vi "Reshape volume imaging data.vi"(0 "tdms file ref":refnum<k34>, 1 "TDMS file path & name":path=path "C:/Users/Theo/Desktop/Datasets/140401_17_44_08-rig 3 debugging/Functional imaging TDMS data files/001.tdms", 5 "All header parameters":T1={"LOGIN"={"User"="Olympus  20X", "Profile"="", "Software Version"="", "Experiment Date Time"=timestamp(0 s since 1904-01-01)}, "GLOBAL PARAMETERS"={"MicroscopeID"="", "Microscope Type"="", "Objective"="", "Field of View (um)"=0.0, "Fill time (us)"=0.0, "Experiment Type"=enum."In vivo", "Stimuli Trigger"=FALSE, "Speed Logging"=FALSE}, "IMAGING MODES"={"Time Series"=FALSE, "Motor Zstack"=FALSE, "AOL Zstack"=FALSE, "Functional Imaging"=FALSE, "Volume Imaging"=FALSE}, "TIME SERIES"={"Basic Image meta data"={"Wavelength (nm)"=0.0, "# averaged frames"=0.0, "laser power (%)"=0.0, "Pockels"=0.0, "pixel dwell time (us)"=0.0, "pmt 1"=0.0, "pmt 2"=0.0, "back apperture"=0.0, "zoom"=0.0, "field of view"=0.0, "Frame Size"=0, "AOL x centre"=200.0, "AOL y centre"=0.0, "Stage x position"=0.0, "Stage y position"=0.0, "Stage z position"=0.0}, "AOL z"=0.0}, "MOTOR Z-STACK "={"Hdr Basic Image meta data"={"Wavelength (nm)"=0.0, "# averaged frames"=0.0, "laser power (%)"=0.0, "Pockels"=0.0, "pixel dwell time (us)"=0.0, "pmt 1"=0.0, "pmt 2"=0.0, "back apperture"=0.0, "zoom"=0.0, "field of view"=0.0, "Frame Size"=0, "AOL x centre"=0.0, "AOL y centre"=0.0, "Stage x position"=0.0, "Stage y position"=0.0, "Stage z position"=0.0}, "Z Start"=0.0, "Z Stop"=0.0, "No of Planes"=0, "Laser Power (%) at Z Start"=0.0, "Laser Power (%) at Z Stop"=0.0}, "AOL Z-STACK"={"Hdr Basic Image meta data"={"Wavelength (nm)"=0.0, "# averaged frames"=0.0, "laser power (%)"=0.0, "Pockels"=0.0, "pixel dwell time (us)"=0.0, "pmt 1"=0.0, "pmt 2"=0.0, "back apperture"=0.0, "zoom"=0.0, "field of view"=0.0, "Frame Size"=0, "AOL x centre"=0.0, "AOL y centre"=0.0, "Stage x position"=0.0, "Stage y position"=0.0, "Stage z position"=0.0}, "Z Start"=0.0, "Z Stop"=0.0, "No of Planes"=0, "Laser Power (%) at Z Start"=0.0, "Laser Power (%) at Z Stop"=0.0}, "FUNCTIONAL IMAGING"={"Functional Mode"=enum."Point", "Variable Length"=FALSE, "Variable Resolution"=FALSE, "Pockels Modulation"=FALSE, "Stimuli Trigger"=FALSE, "Cool down enabled"=FALSE, "AOL Mode"=enum."Raster", "Plane Mode"=0, "Miniscan Dwell time per pixel (us)"=0.0, "poi dwell time"=0.0, "Number of trials"=0.0, "Number of cycles"=0.0, "Number of pois"=0.0, "Number of miniscans"=0.0, "Number of pixels in miniscan"=0.0, "Rectangle ROI length"=0.0, "Rectangle ROI height"=0.0, "Frame rate (fps)"=0.0, "Acquisition Length"=0.0, "video length (sec)"=0.0, "Stimuli delay (sec)"=0.0, "Cool down time (sec)"=0.0, "Basic Image meta data"={"Wavelength (nm)"=0.0, "# averaged frames"=0.0, "laser power (%)"=0.0, "Pockels"=0.0, "pixel dwell time (us)"=0.0, "pmt 1"=0.0, "pmt 2"=0.0, "back apperture"=0.0, "zoom"=0.0, "field of view"=0.0, "Frame Size"=0, "AOL x centre"=0.0, "AOL y centre"=0.0, "Stage x position"=0.0, "Stage y position"=0.0, "Stage z position"=0.0}, "Z Start (um)"=0.0, "Z Stop (um)"=0.0}, "VOLUME IMAGING"={"Functional Mode"=enum."Point", "Variable Length"=FALSE, "Variable Resolution"=FALSE, "Pockels Modulation"=FALSE, "Stimuli Trigger"=FALSE, "Cool down enabled"=FALSE, "AOL Mode"=enum."Raster", "Plane Mode"=0, "Miniscan Dwell time per pixel (us)"=0.0, "poi dwell time"=0.0, "Number of trials"=0.0, "Number of cycles"=0.0, "Number of pois"=0.0, "Number of miniscans"=0.0, "Number of pixels in miniscan"=0.0, "Rectangle ROI length"=0.0, "Rectangle ROI height"=0.0, "Frame rate (fps)"=0.0, "Acquisition Length"=0.0, "video length (sec)"=0.0, "Stimuli delay (sec)"=0.0, "Cool down time (sec)"=0.0, "Basic Image meta data"={"Wavelength (nm)"=0.0, "# averaged frames"=0.0, "laser power (%)"=0.0, "Pockels"=0.0, "pixel dwell time (us)"=0.0, "pmt 1"=0.0, "pmt 2"=0.0, "back apperture"=0.0, "zoom"=0.0, "field of view"=0.0, "Frame Size"=0, "AOL x centre"=0.0, "AOL y centre"=0.0, "Stage x position"=0.0, "Stage y position"=0.0, "Stage z position"=0.0}, "Z Start (um)"=0.0, "Z Stop (um)"=0.0}, "MOVEMENT CORRECTION"={"Movement Correction"=FALSE, "Axial Reference"=FALSE, "Reference Source"=enum."Green channel", "Full Frame Size"=0.0, "Reference Field of View"=0.0, "Reference Zoom"=0.0, "Reference dwell time (us)"=0.0, "Reference X Pixels"=0.0, "Reference Y Pixels"=0.0, "Number of Z lines"=0.0, "Size of Z pixels"=0.0, "Axial Pixels"=0.0, "Ignore Z lines"=0.0, "Reference Scan Cycles"=0.0, "Reference Threshold XY"=0.0, "Reference Threshold Z"=0.0, "Reference Average XY"=0.0, "Reference Average Z"=0.0, "Proportional Scale"=0.0, "Integral Scale"=0.0, "Proportional Scale Z"=0.0, "Integral Scale Z"=0.0, "Diff Threshold"=0.0, "Diff Threshold Z"=0.0, "Sliding Average"=FALSE, "Reference count reset enabled"=FALSE, "Scan Interval (ms)"=0.0, "Ref Plot Refresh Rate (ms)"=0.0}, "CALIBRATION"={"Pockels Calibration File"=path "", "Calibration_ini file"=path "", "Setup_ini file"=path ""}, "STATISTICS"={"Z-stack duration (sec)"=0.0, "Number of acquired data-points"=0.0, "Acquisition time (ms)"=0.0, "Number of acquired frames"=0.0, "Intertrial times"=[]}, "BIOLOGY INFORMATION"={"Animal Code or Name"="", "Animal DoB"="", "Animal Age"="", "Animal Sex"="", "Animal Weight"="", "Date of Injection"="", "Date of Implant"="", "Site of Injection"="", "Animal Ear Notch"="", "AAV constructs"="", "Genetic background"="", "Optical reporter"="", "Region of brain imaged"="", "Other \ncomments"=""}, "Calibration Data"={"Objective Name"="", "Calibration Wavelength"=0.0, "Sum X"=0.0, "Sum Y"=0.0, "Diff X"=0.0, "Diff Y"=0.0, "Distortion Correction"=0.0, " Z norm to um Scaling"=0.0, " X norm to um Scaling"=0.0}} {"VOLUME IMAGING"."Plane Mode" items=["XY Plane", "XZ Plane", "YZ Plane", "arbitraryplane"]; "VOLUME IMAGING"."Basic Image meta data"."Frame Size" items=["100X100"=100, "128X128"=128, "200X200"=200, "256X256"=256, "512X512"=512, "1024x1024"=1024, "2048x2048"=2048]; "AOL Z-STACK"."Hdr Basic Image meta data"."Frame Size" items=["100X100"=100, "128X128"=128, "200X200"=200, "256X256"=256, "512X512"=512, "1024x1024"=1024, "2048x2048"=2048]; "MOTOR Z-STACK"."Hdr Basic Image meta data"."Frame Size" items=["100X100"=100, "128X128"=128, "200X200"=200, "256X256"=256, "512X512"=512, "1024x1024"=1024, "2048x2048"=2048]; "FUNCTIONAL IMAGING"."Plane Mode" items=["XY Plane", "XZ Plane", "YZ Plane", "arbitraryplane"]; "FUNCTIONAL IMAGING"."Basic Image meta data"."Frame Size" items=["100X100"=100, "128X128"=128, "200X200"=200, "256X256"=256, "512X512"=512, "1024x1024"=1024, "2048x2048"=2048]; "TIME SERIES"."Basic Image meta data"."Frame Size" items=["100X100"=100, "128X128"=128, "200X200"=200, "256X256"=256, "512X512"=512, "1024x1024"=1024, "2048x2048"=2048]}, 11 "error in (no error)":errorcluster, 12 "Channel to process":enum16{"Red", "Green", "Both"}(ring)) -> (4 "tdms file out":refnum<k34>, 6 "Single channel data":u16[](array[numeric]), 8 "Channel 4D data":u16[][][][](array[numeric]), 10 "Volumetric parameters":T21, 14 "Angles (deg)":dbl[](array[numeric]), 15 "error out":errorcluster)   [LabVIEW 2020]
uses:
  User Interface/Visualisation/Functional Imaging Viewer/SubVIs/Experiment header interface/Typedefs/Header parameters cluster-ALL.ctl
  User Interface/Visualisation/Functional Imaging Viewer/SubVIs/Experiment header interface/Typedefs/Header subclusters/Header params -Login.ctl
  User Interface/Visualisation/Functional Imaging Viewer/SubVIs/Experiment header interface/Typedefs/Header subclusters/Header params-Global Parameters.ctl
  User Interface/Misc/Experiment Type.ctl
  User Interface/Visualisation/Functional Imaging Viewer/SubVIs/Experiment header interface/Typedefs/Header subclusters/Header params-Imaging Modes.ctl
  User Interface/Visualisation/Functional Imaging Viewer/SubVIs/Experiment header interface/Typedefs/Header subclusters/Header params-Time Series.ctl
  User Interface/Visualisation/Functional Imaging Viewer/SubVIs/Experiment header interface/Typedefs/Header subclusters/Header params-Basic image meta data.ctl
  Typedefs/Frame Size.ctl
  User Interface/Visualisation/Functional Imaging Viewer/SubVIs/Experiment header interface/Typedefs/Header subclusters/Header params-Motor Z-stack.ctl
  User Interface/Visualisation/Functional Imaging Viewer/SubVIs/Experiment header interface/Typedefs/Header subclusters/Header params-AOL Z-stack.ctl
  User Interface/Visualisation/Functional Imaging Viewer/SubVIs/Experiment header interface/Typedefs/Header subclusters/Header params-Functional Imaging.ctl
  Typedefs/Functional Mode.ctl
  Typedefs/AOL modes.ctl
  Typedefs/Plane Mode.ctl
  User Interface/Visualisation/Functional Imaging Viewer/SubVIs/Experiment header interface/Typedefs/Header subclusters/Header params-Movement correction.ctl
  Typedefs/Reference source.ctl
  User Interface/Visualisation/Functional Imaging Viewer/SubVIs/Experiment header interface/Typedefs/Header subclusters/Header params-Calibration Setup.ctl
  User Interface/Visualisation/Functional Imaging Viewer/SubVIs/Experiment header interface/Typedefs/Header subclusters/Header params-statistics.ctl
  User Interface/Misc/Biology Information.ctl
  User Interface/Visualisation/Functional Imaging Viewer/SubVIs/Experiment header interface/Typedefs/Header subclusters/Header params-calibration data.ctl
panel:
  in  "Channel to process":enum16{"Red", "Green"}(ring)
  out "Points in each volume or trial (fractional)":dbl
  out "Points Mismatch":bool
  out "Resulting number of points":i32
  out "Points in each volume or trial":i32
  out "Points in all volumes":i32
  out "Channel size(s)":i32[](array[numeric])
  # "<---This should be an integer. If it is not review the logic inside this VI is suitable"
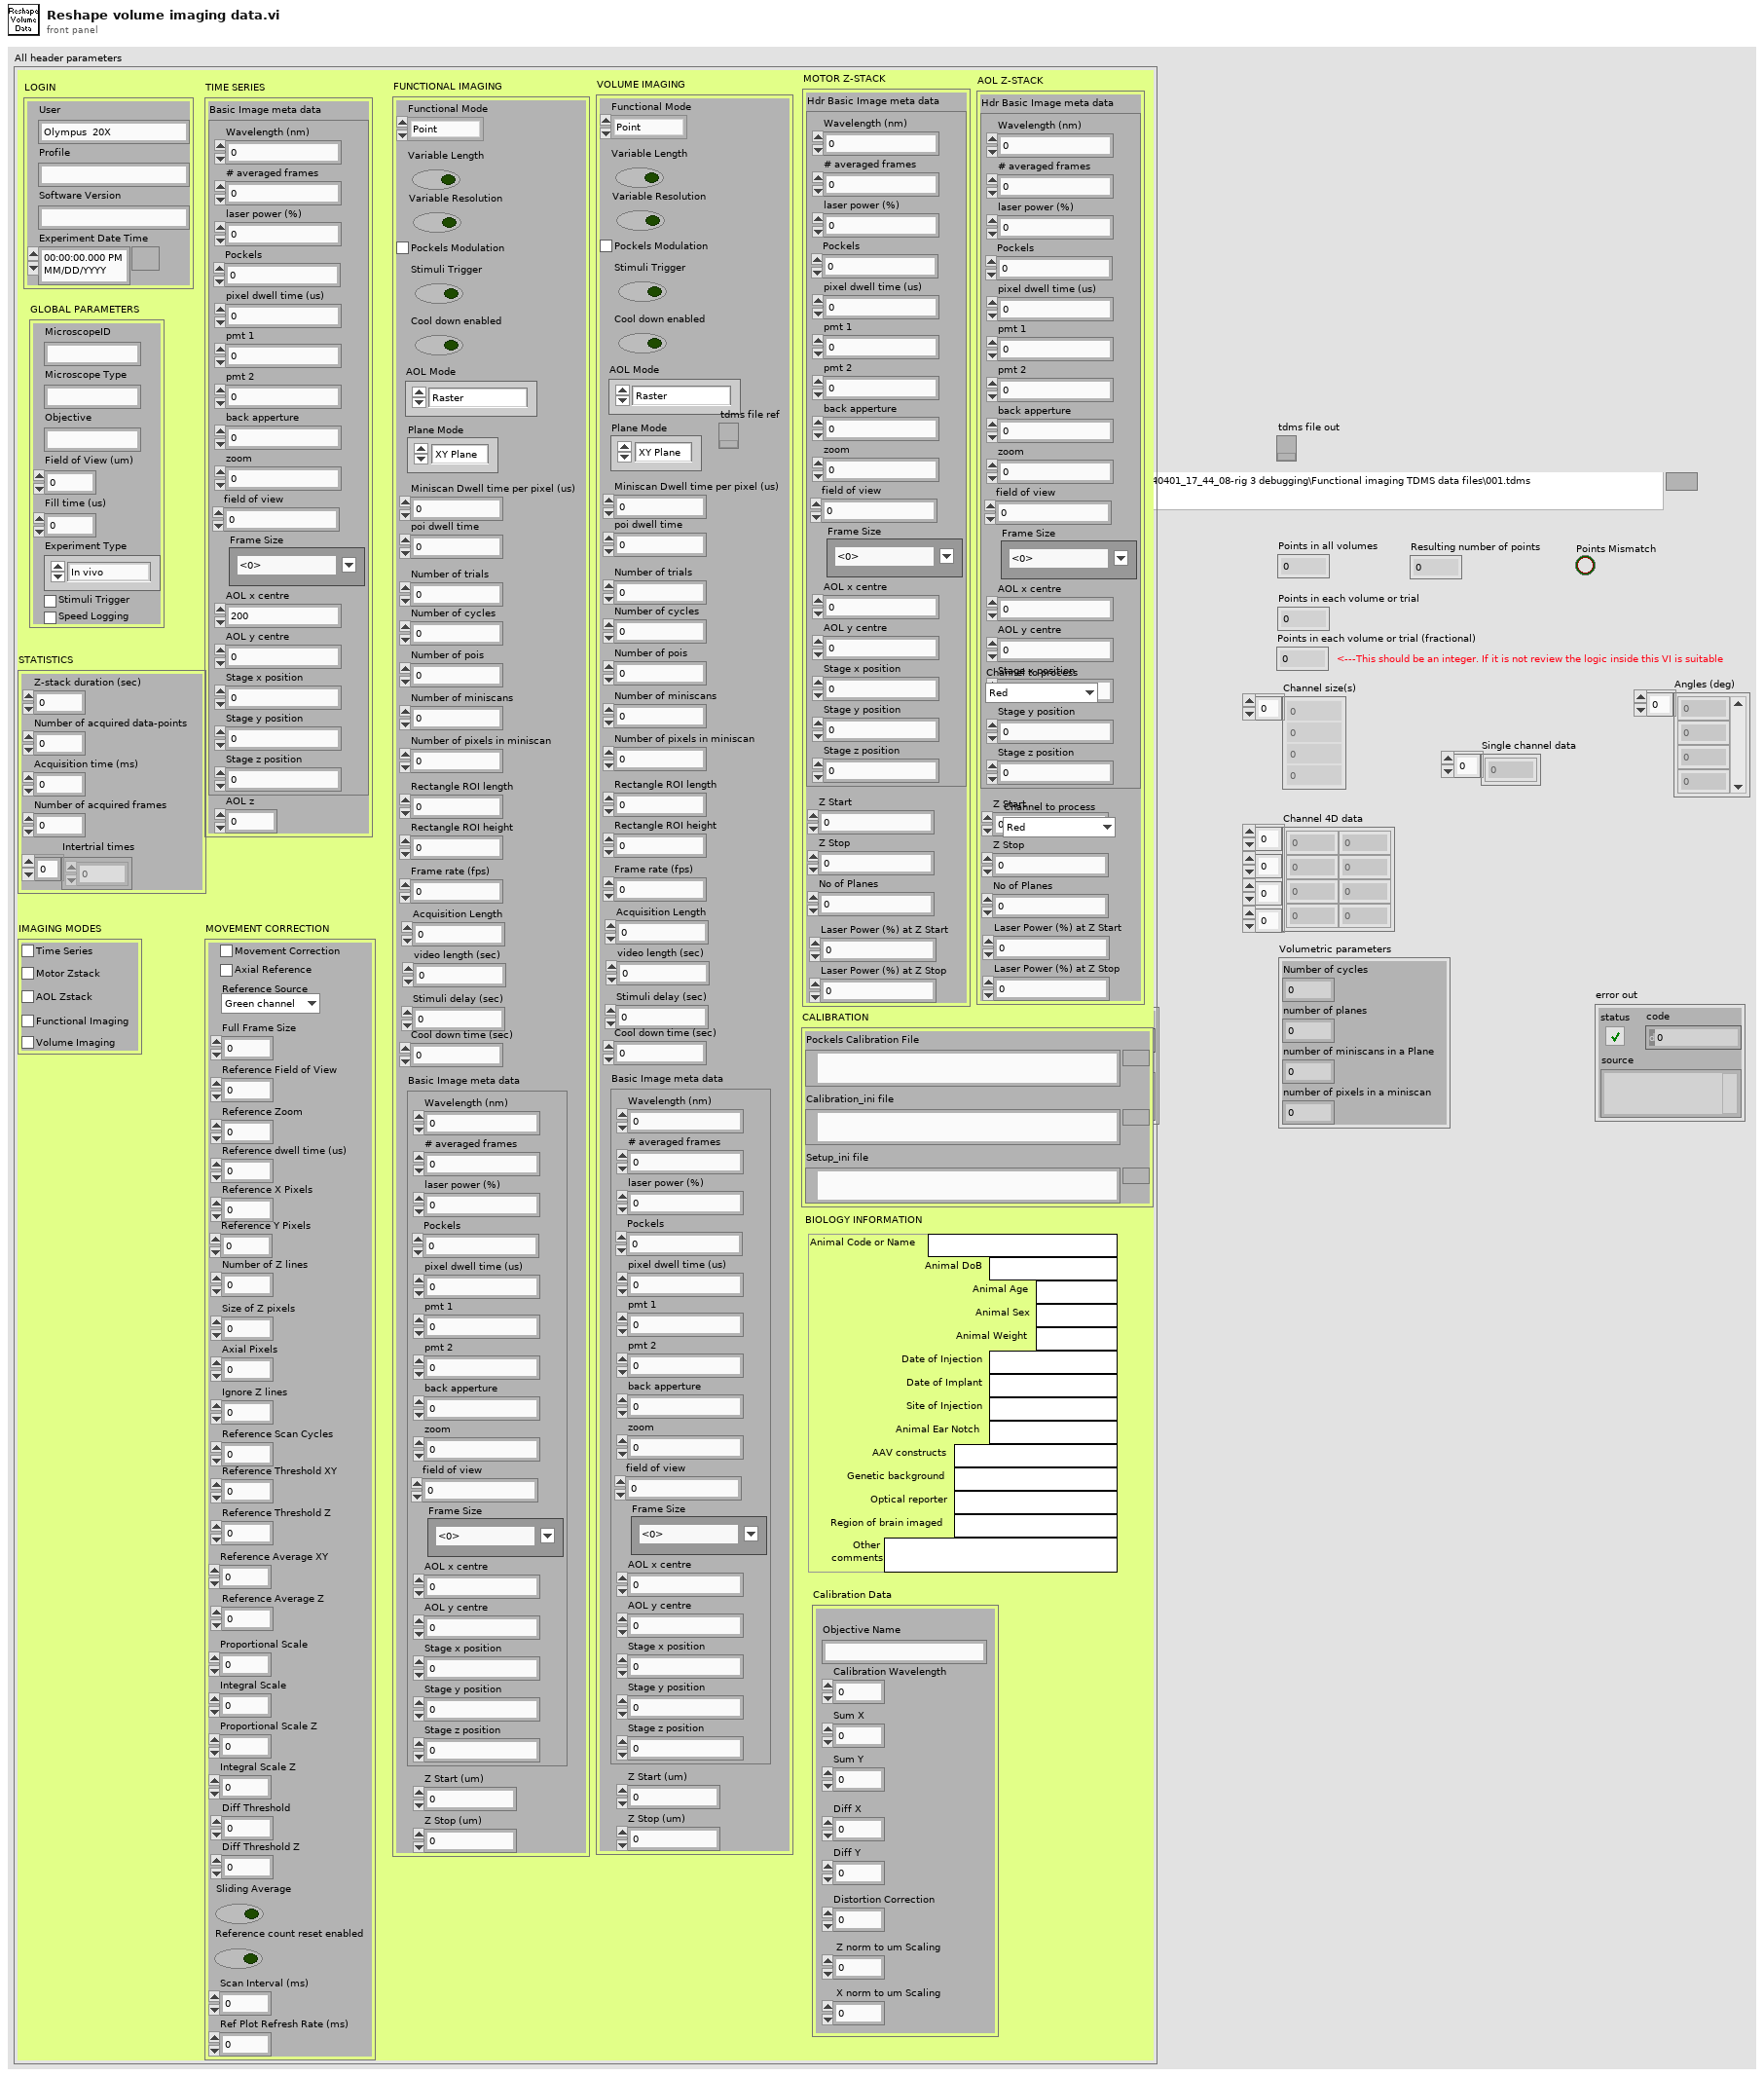
[diagram p1: front panel]
types:
  T1 = typedef "Header parameters cluster-ALL.ctl" = cluster{"LOGIN":T2, "GLOBAL PARAMETERS":T3, "IMAGING MODES":T5, "TIME SERIES":T6, "MOTOR Z-STACK ":T9, "AOL Z-STACK":T10, "FUNCTIONAL IMAGING":T11, "VOLUME IMAGING":T11, "MOVEMENT CORRECTION":T15, "CALIBRATION":T17, "STATISTICS":T18, "BIOLOGY INFORMATION":T19, "Calibration Data":T20}
  T2 = typedef "Header params -Login.ctl" = cluster{"User":string, "Profile":string, "Software Version":string, "Experiment Date Time":timestamp}
  T3 = typedef "Header params-Global Parameters.ctl" = cluster{"MicroscopeID":string, "Microscope Type":string, "Objective":string, "Field of View (um)":dbl, "Fill time (us)":dbl, "Experiment Type":T4, "Stimuli Trigger":bool, "Speed Logging":bool}
  T4 = typedef "Experiment Type.ctl" = enum16{"In vivo", "In vitro", "Testing", "Calibration", "Other"}
  T5 = typedef "Header params-Imaging Modes.ctl" = cluster{"Time Series":bool, "Motor Zstack":bool, "AOL Zstack":bool, "Functional Imaging":bool, "Volume Imaging":bool}
  T6 = typedef "Header params-Time Series.ctl" = cluster{"Basic Image meta data":T7, "AOL z":dbl}
  T7 = typedef "Header params-Basic image meta data.ctl" = cluster{"Wavelength (nm)":dbl, "# averaged frames":dbl, "laser power (%)":dbl, "Pockels":dbl, "pixel dwell time (us)":dbl, "pmt 1":dbl, "pmt 2":dbl, "back apperture":dbl, "zoom":dbl, "field of view":dbl, "Frame Size":T8, "AOL x centre":dbl, "AOL y centre":dbl, "Stage x position":dbl, "Stage y position":dbl, "Stage z position":dbl}
  T8 = typedef "Frame Size.ctl" = u16
  T9 = typedef "Header params-Motor Z-stack.ctl" = cluster{"Hdr Basic Image meta data":T7, "Z Start":dbl, "Z Stop":dbl, "No of Planes":i32, "Laser Power (%) at Z Start":dbl, "Laser Power (%) at Z Stop":dbl}
  T10 = typedef "Header params-AOL Z-stack.ctl" = cluster{"Hdr Basic Image meta data":T7, "Z Start":dbl, "Z Stop":dbl, "No of Planes":i32, "Laser Power (%) at Z Start":dbl, "Laser Power (%) at Z Stop":dbl}
  T11 = typedef "Header params-Functional Imaging.ctl" = cluster{"Functional Mode":T12, "Variable Length":bool, "Variable Resolution":bool, "Pockels Modulation":bool, "Stimuli Trigger":bool, "Cool down enabled":bool, "AOL Mode":T13, "Plane Mode":T14, "Miniscan Dwell time per pixel (us)":dbl, "poi dwell time":dbl, "Number of trials":dbl, "Number of cycles":dbl, "Number of pois":dbl, "Number of miniscans":dbl, "Number of pixels in miniscan":dbl, "Rectangle ROI length":dbl, "Rectangle ROI height":dbl, "Frame rate (fps)":dbl, "Acquisition Length":dbl, "video length (sec)":dbl, "Stimuli delay (sec)":dbl, "Cool down time (sec)":dbl, "Basic Image meta data":T7, "Z Start (um)":dbl, "Z Stop (um)":dbl}
  T12 = typedef "Functional Mode.ctl" = enum16{"Point", "Line", "Patch", "Plane", "Volume"}
  T13 = typedef "AOL modes.ctl" = enum16{"Raster", "Structural", "Pointing", "Mini Scan", "Alignment"}
  T14 = typedef "Plane Mode.ctl" = u16
  T15 = typedef "Header params-Movement correction.ctl" = cluster{"Movement Correction":bool, "Axial Reference":bool, "Reference Source":T16, "Full Frame Size":dbl, "Reference Field of View":dbl, "Reference Zoom":dbl, "Reference dwell time (us)":dbl, "Reference X Pixels":dbl, "Reference Y Pixels":dbl, "Number of Z lines":dbl, "Size of Z pixels":dbl, "Axial Pixels":dbl, "Ignore Z lines":dbl, "Reference Scan Cycles":dbl, "Reference Threshold XY":dbl, "Reference Threshold Z":dbl, "Reference Average XY":dbl, "Reference Average Z":dbl, "Proportional Scale":dbl, "Integral Scale":dbl, "Proportional Scale Z":dbl, "Integral Scale Z":dbl, "Diff Threshold":dbl, "Diff Threshold Z":dbl, "Sliding Average":bool, "Reference count reset enabled":bool, "Scan Interval (ms)":dbl, "Ref Plot Refresh Rate (ms)":dbl}
  T16 = typedef "Reference source.ctl" = enum16{"Green channel", "Red channel"}
  T17 = typedef "Header params-Calibration Setup.ctl" = cluster{"Pockels Calibration File":path, "Calibration_ini file":path, "Setup_ini file":path}
  T18 = typedef "Header params-statistics.ctl" = cluster{"Z-stack duration (sec)":dbl, "Number of acquired data-points":dbl, "Acquisition time (ms)":dbl, "Number of acquired frames":dbl, "Intertrial times":dbl[]}
  T19 = typedef "Biology Information.ctl" = cluster{"Animal Code or Name":string, "Animal DoB":string, "Animal Age":string, "Animal Sex":string, "Animal Weight":string, "Date of Injection":string, "Date of Implant":string, "Site of Injection":string, "Animal Ear Notch":string, "AAV constructs":string, "Genetic background":string, "Optical reporter":string, "Region of brain imaged":string, "Other \ncomments":string}
  T20 = typedef "Header params-calibration data.ctl" = cluster{"Objective Name":string, "Calibration Wavelength":dbl, "Sum X":dbl, "Sum Y":dbl, "Diff X":dbl, "Diff Y":dbl, "Distortion Correction":dbl, " Z norm to um Scaling":dbl, " X norm to um Scaling":dbl}
  T21 = cluster{"Number of cycles":i32, "number of planes":i32, "number of miniscans in a Plane":i32, "number of pixels in a miniscan":i32}
  T22 = cluster{"Number of trials/volumes":i32, "number of planes":i32, "number of miniscans in a Plane":i32, "number of pixels in a miniscan":i32}
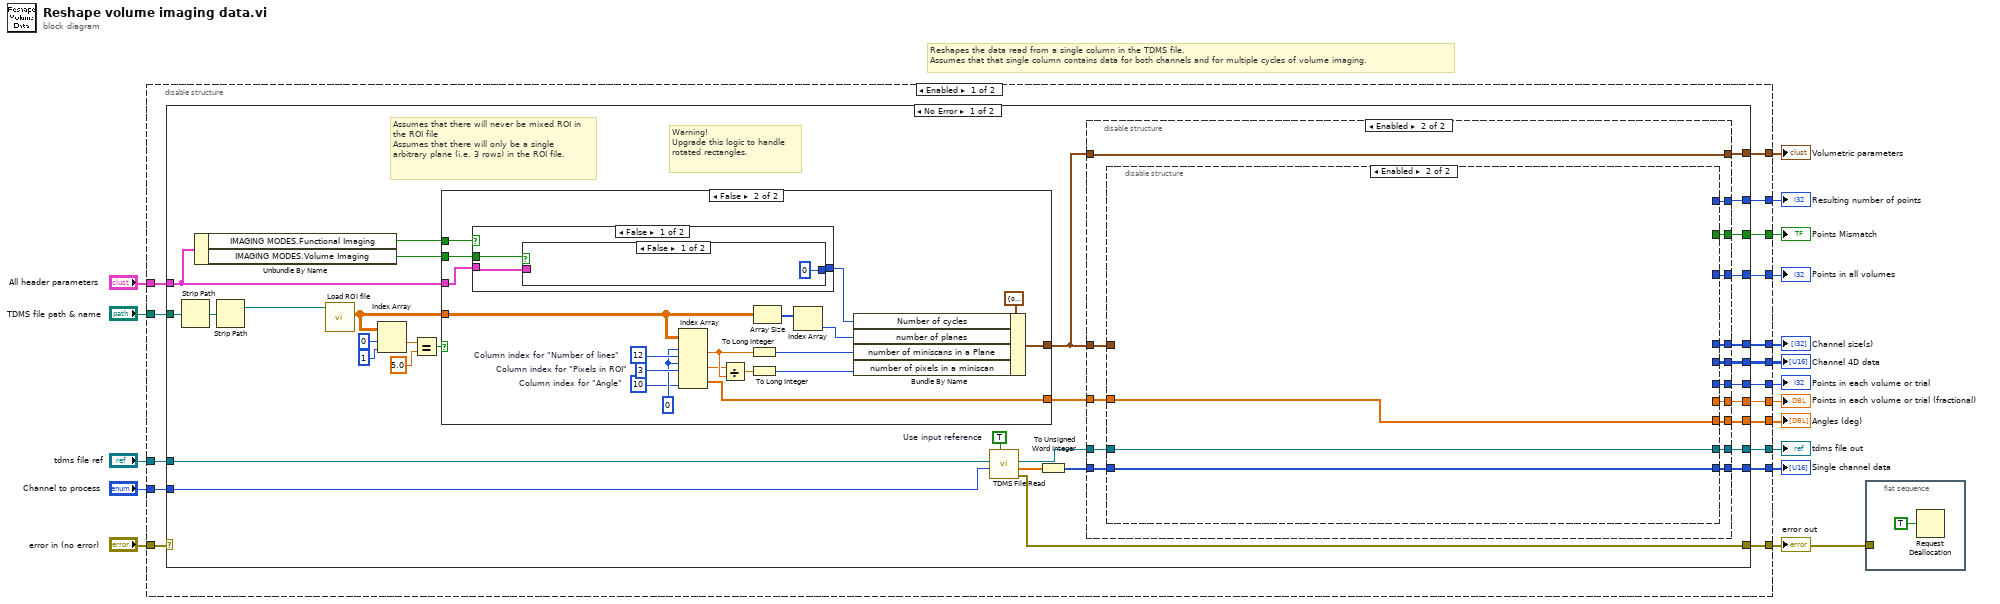
[diagram p0: block diagram]
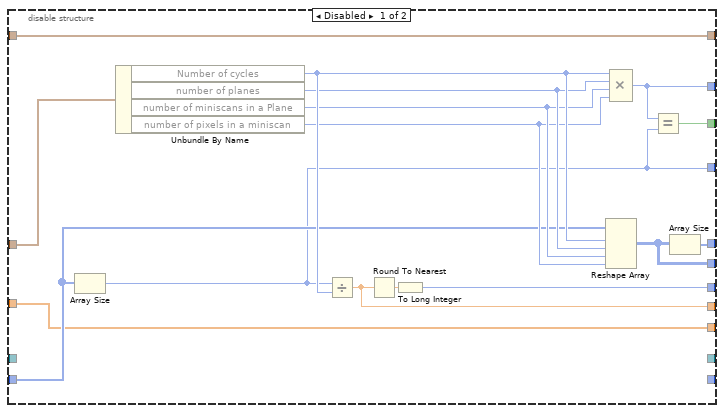
[diagram p2: hidden frame]
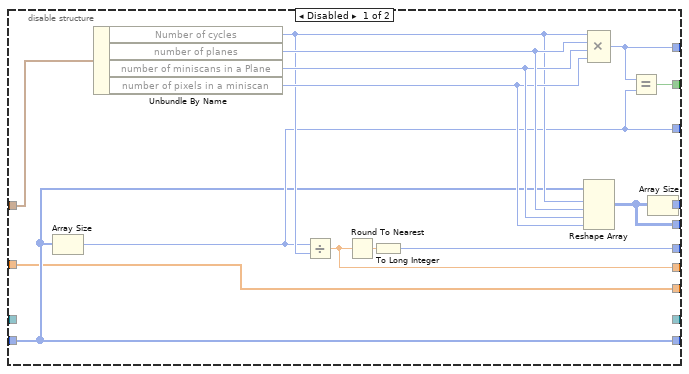
[diagram p3: hidden frame]
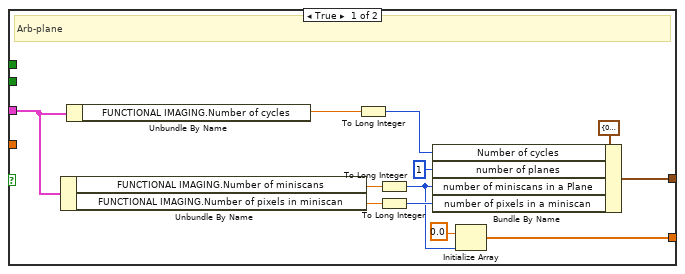
[diagram p4: hidden frame]
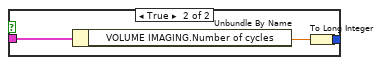
[diagram p5: hidden frame]
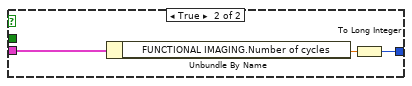
[diagram p6: hidden frame]
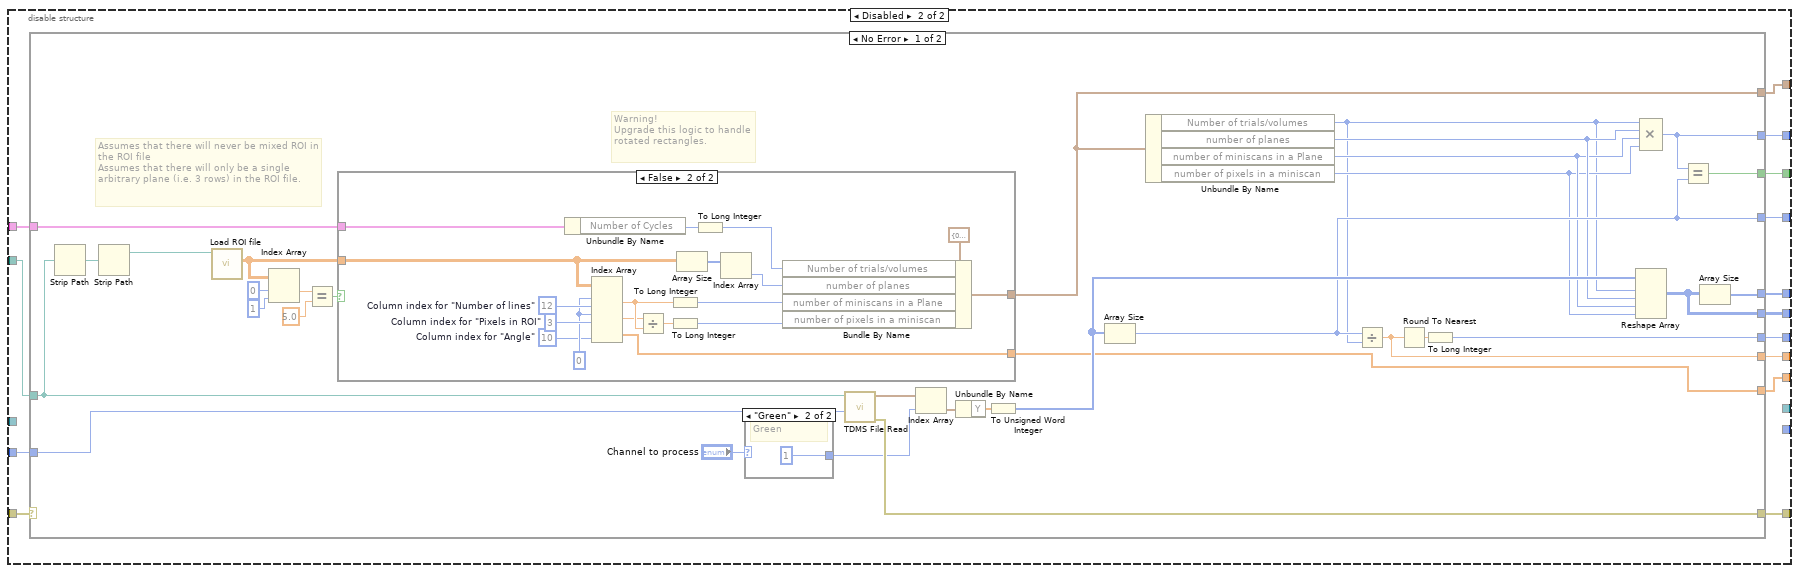
[diagram p8: hidden frame]
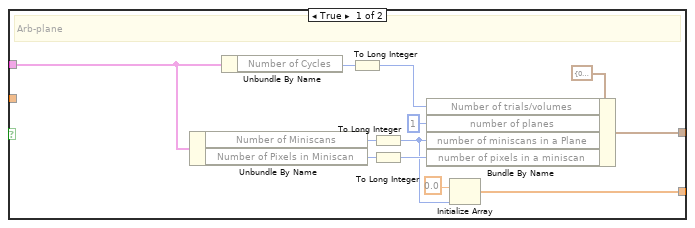
[diagram p9: hidden frame]
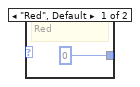
[diagram p10: hidden frame]
diagram:
  # "Reshapes the data read from a single column in the TDMS file.\nAssumes that that single column contains data for both channels and for multiple cycles of volume imaging."
  n1 = disable-structure shown="Enabled" {
    disable-tunnel: [w34 w171] -> w17
    disable-tunnel: "TDMS file path & name" -> [w33 w170]
    disable-tunnel: [w32 w169] -> w15
    disable-tunnel: [w31 w168] -> w14
    disable-tunnel: [w30 w167] -> w13
    disable-tunnel: "error in (no error)" -> [w29 w166]
    disable-tunnel: [w28 w165] -> w11
    disable-tunnel: [w27 w164] -> w10
    disable-tunnel: [w26 w163] -> w9
    disable-tunnel: "All header parameters" -> [w25 w162]
    disable-tunnel: [w24 w161] -> w7
    disable-tunnel: [w23 w160] -> w6
    disable-tunnel: [w22 w159] -> w5
    disable-tunnel: "Channel to process" -> [w21 w158]
    disable-tunnel: [w20 _] -> w3
    disable-tunnel: "tdms file ref" -> [w19 _]
    disable-tunnel: [w18 _] -> w1
    frame Enabled {
      n2 = case shown="No Error" w29 {
        selector: w29 -> [_ w157]
        tunnel: [w66 _] -> w34
        tunnel: w33 -> [w60 _]
        tunnel: [w65 _] -> w32
        tunnel: [w64 _] -> w31
        tunnel: [w63 _] -> w30
        tunnel: [w59 w157] -> w28
        tunnel: w25 -> [w37 _]
        tunnel: [w43 _] -> w26
        tunnel: [w47 _] -> w27
        tunnel: [w51 _] -> w24
        tunnel: [w50 _] -> w23
        tunnel: [w49 _] -> w22
        tunnel: w21 -> [w46 _]
        tunnel: [w45 _] -> w20
        tunnel: w19 -> [w41 _]
        tunnel: [w38 _] -> w18
        frame No Error {
          w42 = TRUE  # Use input reference
          # "Assumes that there will never be mixed ROI in the ROI file\nAssumes that there will only be a single arbitrary plane (i.e. 3 rows) in the ROI file."
          # "Warning!\nUpgrade this logic to handle rotated rectangles."
          n3 = Strip Path(path=w60) -> (stripped path=w61:path)  [unwired: 1 out]
          n4 = Unbundle By Name(w37) -> ("IMAGING MODES.Functional Imaging"=w36:bool, "IMAGING MODES.Volume Imaging"=w35:bool)
          n5 = Strip Path(path=w61) -> (stripped path=w62:path)  [unwired: 1 out]
          n6 = call "Load ROI file.vi"("Experiment data folder path"=w62) -> ("ROI Data (header removed)"=w58:dbl[][])  [unwired: 7 in, 3 out]
          n7 = Index Array(array=w58, index (row)=0, index (col)=1 ("disabled index (col)")) -> (element=w55:dbl)
          n8 = Equal?(x=w55, y=5.0) -> (x = y?=w53:bool)
          n9 = case shown="False" w53 {
            tunnel: [w127 w142] -> w44
            tunnel: [w123 w133] -> w48
            tunnel: w58 -> [_ w134]
            tunnel: w37 -> [w119 w131]
            tunnel: w36 -> [_ w129]
            tunnel: w35 -> [_ w128]
            frame True {
              # "Arb-plane"
              n10 = Unbundle By Name(w119) -> ("FUNCTIONAL IMAGING.Number of miniscans"=w118:dbl, "FUNCTIONAL IMAGING.Number of pixels in miniscan"=w117:dbl)
              n11 = Unbundle By Name(w119) -> ("FUNCTIONAL IMAGING.Number of cycles"=w121:dbl)
              n12 = To Long Integer(number=w121) -> (32bit integer=w120:i32)
              n13 = To Long Integer(number=w118) -> (32bit integer=w122:i32)
              n14 = To Long Integer(number=w117) -> (32bit integer=w125:i32)
              n15 = Bundle By Name(cluster=T21 {"Number of cycles"=0, "number of planes"=0, "number of miniscans in a Plane"=0, "number of pixels in a miniscan"=0} ("Parameters Cluster"), "Number of cycles"=w120, "number of planes"=1, "number of miniscans in a Plane"=w122, "number of pixels in a miniscan"=w125) -> (w127:T21)
              n16 = Initialize Array(0.0 ("element"), w122) -> (w123:dbl[])
            }
            frame False {
              w139 = 10  # Column index for "Angle"
              w140 = 0 ("disabled index (row)")
              w145 = 3  # Column index for "Pixels in ROI"
              w146 = 12  # Column index for "Number of lines"
              n17 = case shown="False" w129 {
                tunnel: [w148 w155] -> w132
                tunnel: w131 -> [w149 w154]
                tunnel: w128 -> [w147 _]
                frame False {
                  n18 = case shown="False" w147 {
                    tunnel: w149 -> [_ w152]
                    tunnel: [0 w151] -> w148
                    frame False {
                    }
                    frame True {
                      n19 = Unbundle By Name(w152) -> ("VOLUME IMAGING.Number of cycles"=w153:dbl)
                      n20 = To Long Integer(number=w153) -> (32bit integer=w151:i32)
                    }
                  }
                }
                frame True {
                  n21 = Unbundle By Name(w154) -> ("FUNCTIONAL IMAGING.Number of cycles"=w156:dbl)
                  n22 = To Long Integer(number=w156) -> (32bit integer=w155:i32)
                }
              }
              n23 = Index Array(array=w134, index (row) #1=w140, index (col) #1=w146, index (row) #2=w140, index (col) #2=w145, index (col) #3=w139) -> (element #1=w138:dbl, element #2=w137:dbl, element #3=w133:dbl[])  [unwired: 1 in]
              n24 = Divide(x=w137, y=w138) -> (x/y=w141:dbl)
              n25 = To Long Integer(number=w138) -> (32bit integer=w136:i32)
              n26 = To Long Integer(number=w141) -> (32bit integer=w135:i32)
              n27 = Array Size(array=w134) -> (size(s)=w144:i32[])
              n28 = Index Array(array=w144) -> (element=w143:i32)  [unwired: 1 in]
              n29 = Bundle By Name(cluster=T21 {"Number of cycles"=0, "number of planes"=0, "number of miniscans in a Plane"=0, "number of pixels in a miniscan"=0} ("Parameters Cluster"), "Number of cycles"=w132, "number of planes"=w143, "number of miniscans in a Plane"=w136, "number of pixels in a miniscan"=w135) -> (w142:T21)
            }
          }
          n30 = call "TDMS File Read.vi"("Use input reference (F)"=w42, "Channel to load"=w46, "tdms file ref"=w41) -> ("Error Out"=w59:errorcluster, "Single channel data"=w40:dbl[], "tdms file out"=w39:refnum<k34>)  [unwired: 4 in, 2 out]
          n31 = To Unsigned Word Integer(number=w40) -> (unsigned 16bit integer=w52:u16[])
          n32 = disable-structure shown="Enabled" {
            disable-tunnel: [w82 w97] -> w66
            disable-tunnel: [w80 w96] -> w65
            disable-tunnel: [w79 w95] -> w64
            disable-tunnel: [w78 w94] -> w63
            disable-tunnel: w44 -> [w67 w90]
            disable-tunnel: w52 -> [w73 w89]
            disable-tunnel: [w72 w93] -> w51
            disable-tunnel: [w71 w92] -> w50
            disable-tunnel: [w70 w91] -> w49
            disable-tunnel: w48 -> [w69 w87]
            disable-tunnel: [w69 w86] -> w47
            disable-tunnel: [_ w88] -> w45
            disable-tunnel: w44 -> [w68 w85]
            disable-tunnel: [w68 w85] -> w43
            disable-tunnel: w39 -> [_ w84]
            disable-tunnel: [_ w83] -> w38
            frame Disabled {
              n33 = Array Size(array=w73) -> (size(s)=w70:i32)
              n34 = Unbundle By Name(w67) -> ("Number of cycles"=w77:i32, "number of planes"=w76:i32, "number of miniscans in a Plane"=w75:i32, "number of pixels in a miniscan"=w74:i32)
              n35 = Divide(x=w70, y=w77) -> (x/y=w71:dbl)
              n36 = Round To Nearest(number=w71) -> (nearest integer value=w81:dbl)
              n37 = To Long Integer(number=w81) -> (32bit integer=w72:i32)
              n38 = Reshape Array(w73, w77, w76, w75, w74) -> (w78:u16[][][][])
              n39 = Compound Arithmetic op=MULTIPLY(w77, w76, w75, w74) -> (w80:i32)
              n40 = Equal?(x=w80, y=w70) -> (x = y?=w79:bool)
              n41 = Array Size(array=w78) -> (size(s)=w82:i32[])
            }
            frame Enabled {
              n42 = disable-structure shown="Enabled" {
                disable-tunnel: [w112 _] -> w97
                disable-tunnel: [w110 _] -> w96
                disable-tunnel: [w109 _] -> w95
                disable-tunnel: [w108 _] -> w94
                disable-tunnel: [w104 _] -> w93
                disable-tunnel: [w103 _] -> w92
                disable-tunnel: [w101 _] -> w91
                disable-tunnel: w90 -> [w100 _]
                disable-tunnel: w89 -> [w99 w115]
                disable-tunnel: [w99 w115] -> w88
                disable-tunnel: w87 -> [w98 w114]
                disable-tunnel: [w98 w114] -> w86
                disable-tunnel: w84 -> [_ w113]
                disable-tunnel: [_ w113] -> w83
                frame Disabled {
                  n43 = Array Size(array=w99) -> (size(s)=w101:i32)
                  n44 = Unbundle By Name(w100) -> ("Number of cycles"=w102:i32, "number of planes"=w107:i32, "number of miniscans in a Plane"=w106:i32, "number of pixels in a miniscan"=w105:i32)
                  n45 = Divide(x=w101, y=w102) -> (x/y=w103:dbl)
                  n46 = Round To Nearest(number=w103) -> (nearest integer value=w111:dbl)
                  n47 = To Long Integer(number=w111) -> (32bit integer=w104:i32)
                  n48 = Reshape Array(w99, w102, w107, w106, w105) -> (w108:u16[][][][])
                  n49 = Compound Arithmetic op=MULTIPLY(w102, w107, w106, w105) -> (w110:i32)
                  n50 = Equal?(x=w110, y=w101) -> (x = y?=w109:bool)
                  n51 = Array Size(array=w108) -> (size(s)=w112:i32[])
                }
                frame Enabled {
                }
              }
            }
          }
        }
        frame Error {
        }
      }
    }
    frame Disabled {
      n52 = case shown="No Error" w166 {
        selector: w166 -> [_ w236]
        tunnel: [w203 _] -> w171
        tunnel: w170 -> [w194 _]
        tunnel: [w199 _] -> w169
        tunnel: [w198 _] -> w168
        tunnel: [w197 _] -> w167
        tunnel: [w192 w236] -> w165
        tunnel: w162 -> [w184 _]
        tunnel: [w193 _] -> w163
        tunnel: [w179 _] -> w164
        tunnel: [w182 _] -> w161
        tunnel: [w181 _] -> w160
        tunnel: [w180 _] -> w159
        tunnel: w158 -> [w172 _]
        frame No Error {
          # "Assumes that there will never be mixed ROI in the ROI file\nAssumes that there will only be a single arbitrary plane (i.e. 3 rows) in the ROI file."
          # "Warning!\nUpgrade this logic to handle rotated rectangles."
          n53 = Strip Path(path=w194) -> (stripped path=w195:path)  [unwired: 1 out]
          n54 = Strip Path(path=w195) -> (stripped path=w196:path)  [unwired: 1 out]
          n55 = call "Load ROI file.vi"("Experiment data folder path"=w196) -> ("ROI Data (header removed)"=w190:dbl[][])  [unwired: 7 in, 3 out]
          n56 = Index Array(array=w190, index (row)=0, index (col)=1 ("disabled index (col)")) -> (element=w187:dbl)
          n57 = Equal?(x=w187, y=5.0) -> (x = y?=w185:bool)
          n58 = case shown="False" w185 {
            tunnel: [w214 w228] -> w193
            tunnel: [w210 w219] -> w179
            tunnel: w190 -> [_ w220]
            tunnel: w184 -> [w206 w216]
            frame True {
              # "Arb-plane"
              n59 = Unbundle By Name(w206) -> ("Number of Miniscans"=w205:u16, "Number of Pixels in Miniscan"=w204:u16)
              n60 = Unbundle By Name(w206) -> ("Number of Cycles"=w208:u64)
              n61 = To Long Integer(number=w208) -> (32bit integer=w207:i32)
              n62 = To Long Integer(number=w205) -> (32bit integer=w209:i32)
              n63 = To Long Integer(number=w204) -> (32bit integer=w212:i32)
              n64 = Bundle By Name(cluster=T22 {"Number of trials/volumes"=0, "number of planes"=0, "number of miniscans in a Plane"=0, "number of pixels in a miniscan"=0} ("Parameters Cluster"), "Number of trials/volumes"=w207, "number of planes"=1, "number of miniscans in a Plane"=w209, "number of pixels in a miniscan"=w212) -> (w214:T22)
              n65 = Initialize Array(0.0 ("element"), w209) -> (w210:dbl[])
            }
            frame False {
              w225 = 10  # Column index for "Angle"
              w226 = 0 ("disabled index (row)")
              w232 = 3  # Column index for "Pixels in ROI"
              w233 = 12  # Column index for "Number of lines"
              n66 = Unbundle By Name(w216) -> ("Number of Cycles"=w218:u64)
              n67 = Index Array(array=w220, index (row) #1=w226, index (col) #1=w233, index (row) #2=w226, index (col) #2=w232, index (col) #3=w225) -> (element #1=w224:dbl, element #2=w223:dbl, element #3=w219:dbl[])  [unwired: 1 in]
              n68 = Divide(x=w223, y=w224) -> (x/y=w227:dbl)
              n69 = To Long Integer(number=w224) -> (32bit integer=w222:i32)
              n70 = To Long Integer(number=w227) -> (32bit integer=w221:i32)
              n71 = Array Size(array=w220) -> (size(s)=w231:i32[])
              n72 = To Long Integer(number=w218) -> (32bit integer=w217:i32)
              n73 = Index Array(array=w231) -> (element=w230:i32)  [unwired: 1 in]
              n74 = Bundle By Name(cluster=T22 {"Number of trials/volumes"=0, "number of planes"=0, "number of miniscans in a Plane"=0, "number of pixels in a miniscan"=0} ("Parameters Cluster"), "Number of trials/volumes"=w217, "number of planes"=w230, "number of miniscans in a Plane"=w222, "number of pixels in a miniscan"=w221) -> (w228:T22)
            }
          }
          n75 = case shown="\"Green\"" "Channel to process" {
            tunnel: [0 ("index") 1 ("index")] -> w191
            frame "Red", Default {
              # "Red"
            }
            frame "Green" {
              # "Green"
            }
          }
          n76 = call "TDMS File Read.vi"("Channel to load"=w172, "File Path"=w194) -> ("Error Out"=w192:errorcluster, "Data"=w202:waveform(dbl)[])  [unwired: 5 in, 3 out]
          n77 = Index Array(array=w202, index=w191) -> (element=w201:waveform(dbl))
          n78 = Unbundle By Name ("Get Waveform Components")(w201) -> ("Y"=w200:dbl[])
          n79 = To Unsigned Word Integer(number=w200) -> (unsigned 16bit integer=w183:u16[])
          n80 = Array Size(array=w183) -> (size(s)=w180:i32)
          n81 = Unbundle By Name(w193) -> ("Number of trials/volumes"=w174:i32, "number of planes"=w177:i32, "number of miniscans in a Plane"=w176:i32, "number of pixels in a miniscan"=w175:i32)
          n82 = Divide(x=w180, y=w174) -> (x/y=w181:dbl)
          n83 = Round To Nearest(number=w181) -> (nearest integer value=w178:dbl)
          n84 = To Long Integer(number=w178) -> (32bit integer=w182:i32)
          n85 = Reshape Array(w183, w174, w177, w176, w175) -> (w197:u16[][][][])
          n86 = Compound Arithmetic op=MULTIPLY(w174, w177, w176, w175) -> (w199:i32)
          n87 = Equal?(x=w199, y=w180) -> (x = y?=w198:bool)
          n88 = Array Size(array=w197) -> (size(s)=w203:i32[])
        }
        frame Error {
        }
      }
    }
  }
  "Channel size(s)" <- w17
  "Resulting number of points" <- w15
  "Points Mismatch" <- w14
  "Channel 4D data" <- w13
  "error out" <- w11
  "Volumetric parameters" <- w9
  "Angles (deg)" <- w10
  "Points in each volume or trial" <- w7
  "Points in each volume or trial (fractional)" <- w6
  "Points in all volumes" <- w5
  "Single channel data" <- w3
  "tdms file out" <- w1
  n89 = flat-sequence {
    tunnel: w11 -> [_]
    frame #0 {
      n90 = Request Deallocation(TRUE ("flag")) -> ()
    }
  }
